vi "Draw Linear Inverted Pendulum VRML.vi"(2 "Path to WRL file":path, 4 "Height":dbl=38.1 format="%.2f", 5 "Pendulum Color":u32(colorbox)) -> (0 "Scene.New Object":refnum<vi>)   [LabVIEW 2015]
uses:
  <vilib>/picture/3D Picture Control/Object/Create Object (drawable).vi
  <vilib>/picture/3D Picture Control/Object/Create Object (name).vi
  <vilib>/picture/3D Picture Control/Object/Add Object (no reference).vi
  <vilib>/picture/3D Picture Control/NI_3D Picture Control.lvlib
panel:
  out "error out":errorcluster
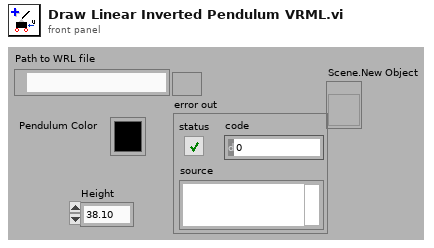
[diagram p1: front panel]
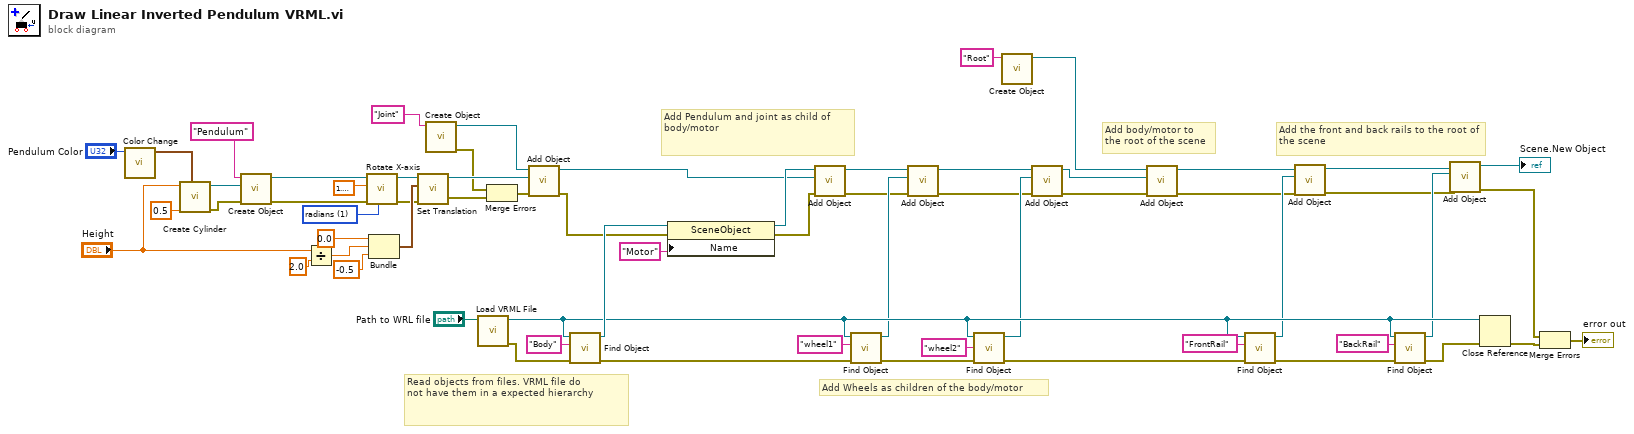
[diagram p0: block diagram]
diagram:
  w16 = u16 1 items=["degree", "radians"] ("angle unit")
  # "Read objects from files. VRML file do\nnot have them in a expected hierarchy"
  # "Add the front and back rails to the root of the scene"
  # "Add body/motor to\nthe root of the scene"
  # "Add Pendulum and joint as child of body/motor"
  # "Add Wheels as children of the body/motor"
  n1 = call <vilib>:"Color Change.vi"("Color"="Pendulum Color") -> ("RGBA"=w59:cluster{"R":sgl, "G":sgl, "B":sgl, "A":sgl})  [unwired: 10 in]
  n2 = call <vilib>:"Create Cylinder.vi"("Color"=w59, "Radius"=sgl 0.5, "Height"="Height") -> ("error out"=w17:errorcluster, "New Cylinder Refnum"=w34:refnum<vi>)  [unwired: 7 in]
  n3 = call-poly <vilib>:"Create Object.vi"("error in (no error)"=w17, "Geometry"=w34, "Name"="Pendulum") -> ("error out"=w15:errorcluster, "Scene:New Object"=w33:refnum<vi>)  [unwired: 7 in]
  n4 = Divide(x="Height", y=2.0) -> (x/y=w52:dbl)
  n5 = call <vilib>:"Rotate X-axis.vi"("angle unit"=w16, "error in (no error)"=w15, "angle"=1.5707963267948966, "Scene Object In"=w33) -> ("error out"=w14:errorcluster, "Scene Object Out"=w61:refnum<vi>)  [unwired: 6 in]
  n6 = Bundle(0.0, w52, -0.5) -> (w54:cluster{dbl, dbl, dbl})  [unwired: 1 in]
  n7 = call <vilib>:"Set Translation.vi"("error in (no error)"=w14, "Translation"=w54, "Scene Object"=w61) -> ("error out"=w11:errorcluster, "Translated Object"=w30:refnum<vi>)  [unwired: 7 in]
  n8 = call-poly <vilib>:"Create Object.vi"("Name"="Joint") -> ("error out"=w10:errorcluster, "Scene:New Object"=w60:refnum<vi>)  [unwired: 9 in]
  n9 = call <vilib>:"Load VRML File.vi"("Path"="Path to WRL file") -> ("error out"=w35:errorcluster, "Scene:Read Scene File"=w36:refnum<vi>)  [unwired: 9 in]
  n10 = Merge Errors(w10, w11) -> (w9:errorcluster)
  n11 = call-poly <vilib>:"Add Object.vi"("error in (no error)"=w9, "New Object In"=w30, "Scene Object In"=w60) -> ("error out"=w2:errorcluster, "Scene Object Out"=w28:refnum<vi>)  [unwired: 7 in]
  n12 = call <vilib>:"Find Object.vi"("error in (no error)"=w35, "Object Name"="Body", "Scene Refnum"=w36) -> ("error out"=w46:errorcluster, "Object Refnum"=w48:refnum<vi>)  [unwired: 7 in]
  n13 = property class="SceneObject"(reference=w48, error in=w2, "Name"="Motor") -> (reference out=w29:refnum<vi>, error out=w1:errorcluster)
  n14 = call-poly <vilib>:"Add Object.vi"("error in (no error)"=w1, "New Object In"=w28, "Scene Object In"=w29) -> ("error out"=w13:errorcluster, "Scene Object Out"=w27:refnum<vi>)  [unwired: 7 in]
  n15 = call <vilib>:"Find Object.vi"("error in (no error)"=w46, "Object Name"="wheel1", "Scene Refnum"=w36) -> ("error out"=w45:errorcluster, "Object Refnum"=w26:refnum<vi>)  [unwired: 7 in]
  n16 = call-poly <vilib>:"Add Object.vi"("error in (no error)"=w13, "New Object In"=w26, "Scene Object In"=w27) -> ("error out"=w12:errorcluster, "Scene Object Out"=w38:refnum<vi>)  [unwired: 7 in]
  n17 = call <vilib>:"Find Object.vi"("error in (no error)"=w45, "Object Name"="wheel2", "Scene Refnum"=w36) -> ("error out"=w43:errorcluster, "Object Refnum"=w25:refnum<vi>)  [unwired: 7 in]
  n18 = call-poly <vilib>:"Create Object.vi"("Name"="Root") -> ("Scene:New Object"=w24:refnum<vi>)  [unwired: 9 in, 1 out]
  n19 = call-poly <vilib>:"Add Object.vi"("error in (no error)"=w12, "New Object In"=w25, "Scene Object In"=w38) -> ("error out"=w8:errorcluster, "Scene Object Out"=w23:refnum<vi>)  [unwired: 7 in]
  n20 = call-poly <vilib>:"Add Object.vi"("error in (no error)"=w8, "New Object In"=w23, "Scene Object In"=w24) -> ("error out"=w7:errorcluster, "Scene Object Out"=w22:refnum<vi>)  [unwired: 7 in]
  n21 = call <vilib>:"Find Object.vi"("error in (no error)"=w43, "Object Name"="FrontRail", "Scene Refnum"=w36) -> ("error out"=w42:errorcluster, "Object Refnum"=w21:refnum<vi>)  [unwired: 7 in]
  n22 = call-poly <vilib>:"Add Object.vi"("error in (no error)"=w7, "New Object In"=w21, "Scene Object In"=w22) -> ("error out"=w6:errorcluster, "Scene Object Out"=w20:refnum<vi>)  [unwired: 7 in]
  n23 = call <vilib>:"Find Object.vi"("error in (no error)"=w42, "Object Name"="BackRail", "Scene Refnum"=w36) -> ("error out"=w37:errorcluster, "Object Refnum"=w19:refnum<vi>)  [unwired: 7 in]
  n24 = call-poly <vilib>:"Add Object.vi"("error in (no error)"=w6, "New Object In"=w19, "Scene Object In"=w20) -> ("error out"=w4:errorcluster, "Scene Object Out"=→"Scene.New Object":refnum<vi>)  [unwired: 7 in]
  n25 = Close Reference(reference=w36, error in (no error)=w37) -> (error out=w5:errorcluster)
  n26 = Merge Errors(w4, w5) -> (→"error out":errorcluster)
